vi "Chirp_EIS_Calculation_deductBias.vi"(8 "error in (no error)":errorcluster, 11 "ChirpEIS in":refnum<class "ChirpEIS.lvclass">) -> (0 "error out":errorcluster, 1 "EIS Results":string, 2 "Show EIS Results":dbl[][](array[numeric]), 3 "ChirpEIS out":refnum<class "ChirpEIS.lvclass">)   [LabVIEW 2014]
uses:
  <vilib>/Analysis/NI_AALPro.lvlib
  <vilib>/Analysis/2dsp.llb/Real FFT.vi
  ChirpEIS.lvclass
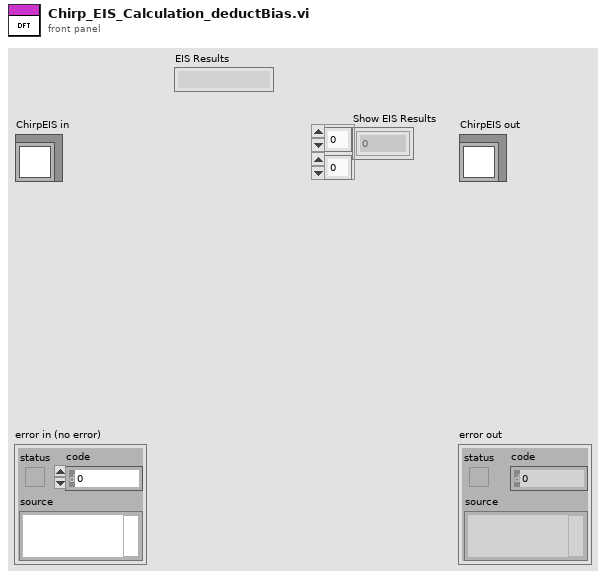
[diagram p1: front panel]
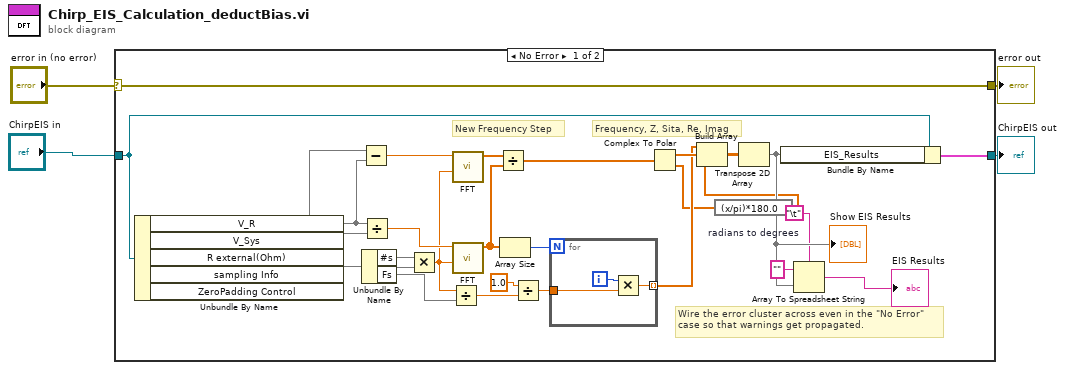
[diagram p0: block diagram]
diagram:
  n1 = case shown="No Error" "error in (no error)" {
    selector: "error in (no error)" -> [w33 w38]
    tunnel: [w33 w38] -> w3
    tunnel: [w11 w37] -> w1
    tunnel: "ChirpEIS in" -> [w12 w37]
    frame No Error {
      # "Frequency, Z, Sita, Re, Imag"
      # "New Frequency Step"
      # "Wire the error cluster across even in the \"No Error\"\ncase so that warnings get propagated."
      n2 = Unbundle By Name(w12) -> ("V_R"=w16, "V_Sys"=w15, "R external(Ohm)"=w13, "sampling Info"=w17, "ZeroPadding Control"=w14)
      n3 = Subtract(x=w15, y=w16) -> (x-y=w32:dbl)
      n4 = Divide(x=w16, y=w13) -> (x/y=w28:dbl)
      n5 = Unbundle By Name(w17) -> ("#s"=w18, "Fs"=w19)
      n6 = Multiply(x=w18, y=w14) -> (x*y=w27:dbl)
      n7 = Divide(x=w27, y=w19) -> (x/y=w20:dbl)
      n8 = call-poly <vilib>:"FFT.vi"("FFT size"=w27, "X"=w32) -> ("FFT {X}"=w29:cdb[])  [unwired: 8 in, 1 out]
      n9 = call-poly <vilib>:"FFT.vi"("FFT size"=w27, "X"=w28) -> ("FFT {X}"=w30:cdb[])  [unwired: 8 in, 1 out]
      n10 = Divide(x=w29, y=w30) -> (x/y=w31:cdb[])
      n11 = Array Size(array=w30) -> (size(s)=w23:i32)
      n12 = Divide(x=1.0, y=w20) -> (x/y=w22:dbl)
      n13 = for {
        N: w23 -> [_]
        tunnel: w22 -> [w36]
        tunnel: [w34] -> w24 mode=indexing
        i -> [w35]
        n14 = Multiply(x=w35, y=w36) -> (x*y=w34:dbl)
      }
      n15 = Complex To Polar(r * e^(i*theta)=w31) -> (r=w25:dbl[], theta=w6:dbl[])
      n16 = expression code="(x/pi)*180.0" "radians to degrees"(w6) -> (w5:dbl[])
      n17 = Build Array(w24, w25, w5) -> (w26:dbl[][])
      n18 = Transpose 2D Array(2D array=w26) -> (transposed array=w10:dbl[][])
      "Show EIS Results" <- w10
      n19 = Bundle By Name(cluster=w12, "EIS_Results"=w10) -> (w11:cluster{})
      n20 = Array To Spreadsheet String(delimiter (Tab)="\t", array=w10, 3:"" ("format string")) -> (spreadsheet string=→"EIS Results":string)
    }
    frame Error {
    }
  }
  "error out" <- w3
  "ChirpEIS out" <- w1
